vi "EOL station.vi"(0 "configuration file path":path caption="配置文件的路径", 1 "EOL station msic inf":T1) -> ()   [LabVIEW 2018]
uses:
  Ctl.xio/EOL station msic ctl.ctl
  SubVIS.xio/DataSocket/DataSocket_Tags.ctl
  Ctl.xio/part type.ctl
  SubVIS.xio/Creat Write List VI's/DefCtrl/Station.ctl
  <vilib>/Utility/file.llb/Read From Spreadsheet File (string).vi
  SubVIS.xio/DataSocket/Read PLC Vars/Read Bool Var.vi
  SubVIS.xio/DataSocket/Read PLC Vars/Read U32 Var.vi
  SubVIS.xio/DataSocket/Write PLC Vars/Write Bool Var in.vi
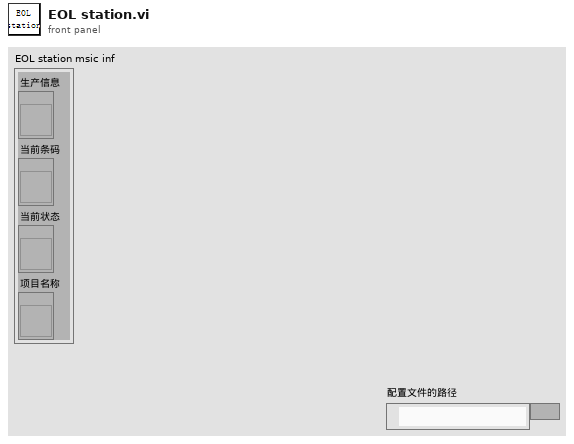
[diagram p1: front panel]
types:
  T1 = cluster{"生产信息":refnum<vi>, "当前条码":refnum<vi>, "当前状态":refnum<vi>, "项目名称":refnum<vi>}
  T2 = typedef "Station.ctl" = enum16{"粗切工位", "热处理工位", "精切工位", "PDF焊接工位", "打凹点预载力工位", "收卷工位", "EOL工位"}
  T3 = typedef "EOL station msic ctl.ctl" = cluster{"configuration file path":path, "DsOut":T4[], "Hopper car information":cluster{"Hopper car code":string, "Hopper car No":string, "plate No":string}, "pallet.produced number":i32, "SQL information":string, "Serial number":i32, "database path":path, "EOL station msic inf":cluster{"生产信息":refnum<vi>, "当前条码":refnum<vi>, "当前状态":refnum<vi>, "项目名称":refnum<vi>}, "part type":T5, "BarCode":string, "scanner resource name out":refnum<visa-resource-name>, "scanner coms":string, "Force value database":string[], "Force value buffer":dbl[], "SN":string, "print inf":string, "2Dcode inf":string, "Pass/Fail":bool}
  T4 = typedef "DataSocket_Tags.ctl" = cluster{"Ds ID":refnum<k13>, "Tag":string}
  T5 = typedef "part type.ctl" = cluster{"Part type":string, "Material code":string, "Part number":string, "Supplier code":string, "Line code":string, "Customer code":string, "Color code":string, "Upper limit":i32, "Temperature":string, "Tot time":string, "EOL stations":string}
  T6 = cluster{"Hopper car code":string, "Hopper car No":string, "plate No":string}
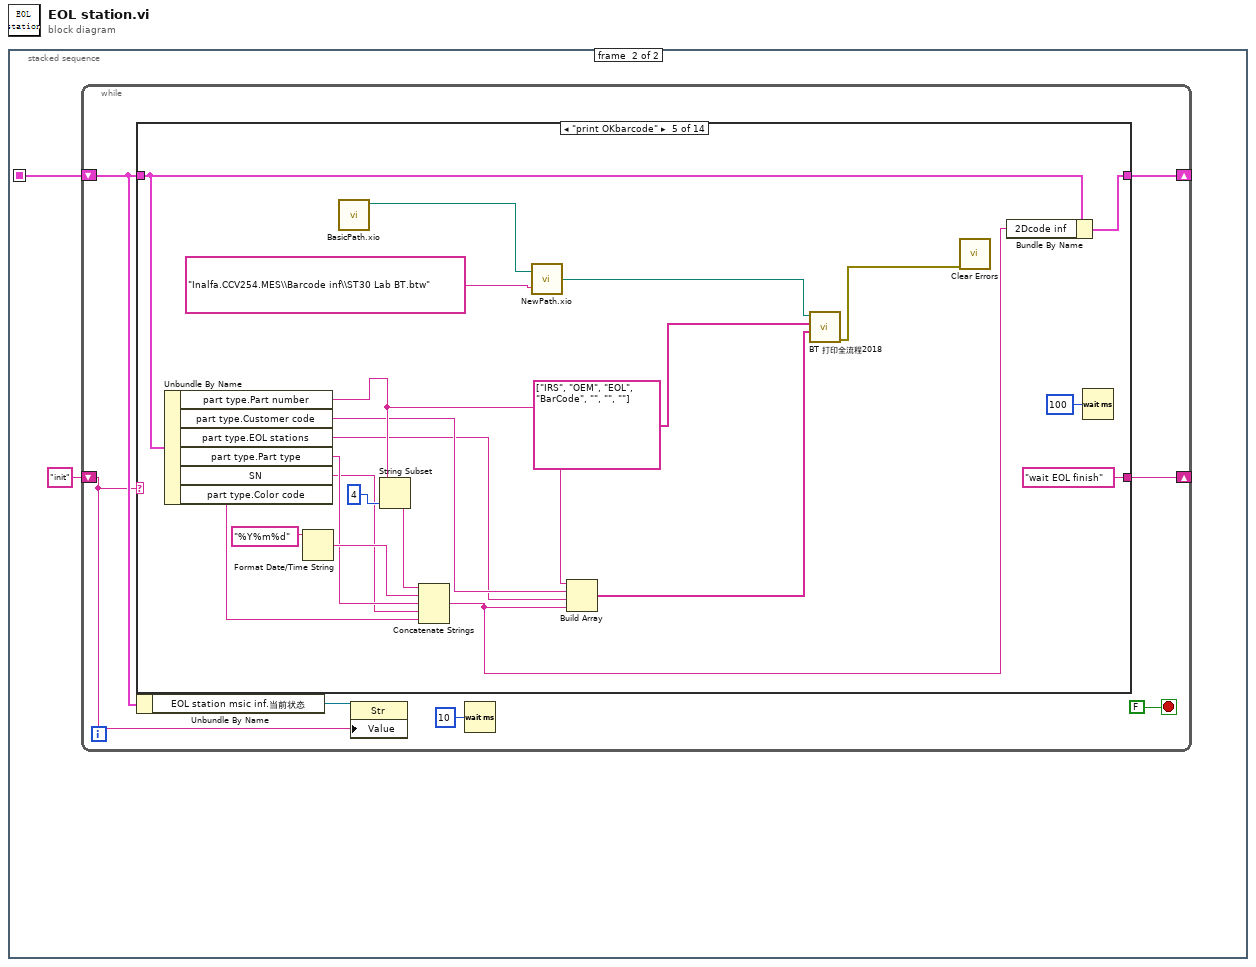
[diagram p0: block diagram]
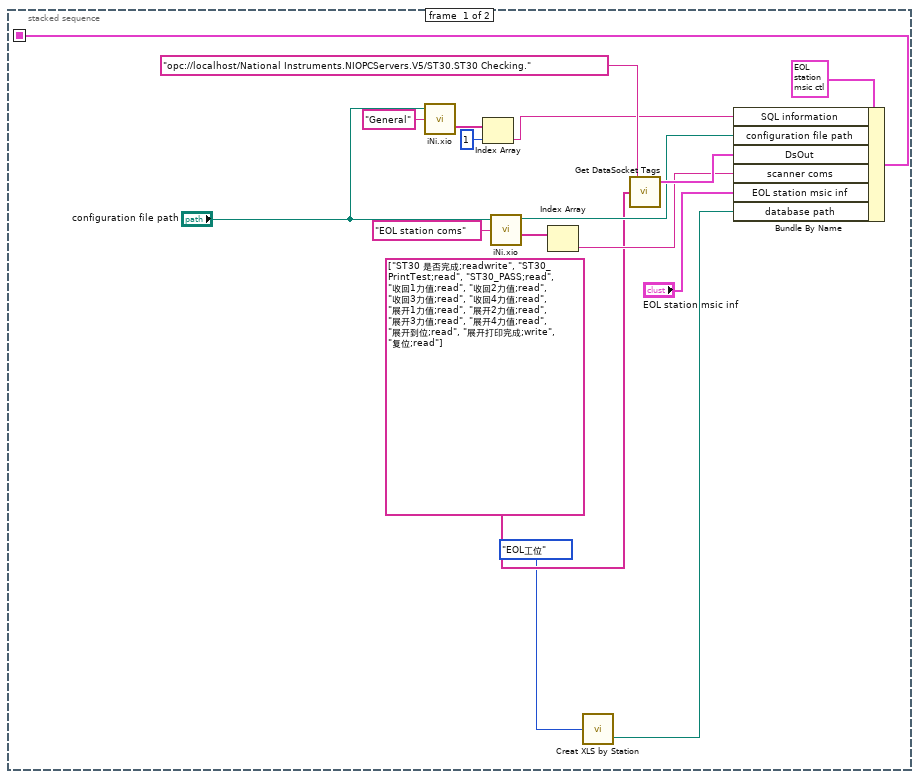
[diagram p2: hidden frame]
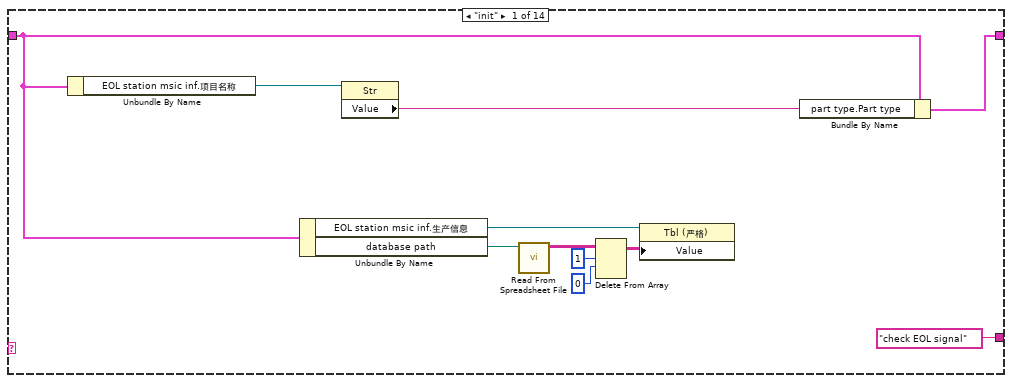
[diagram p3: hidden frame]
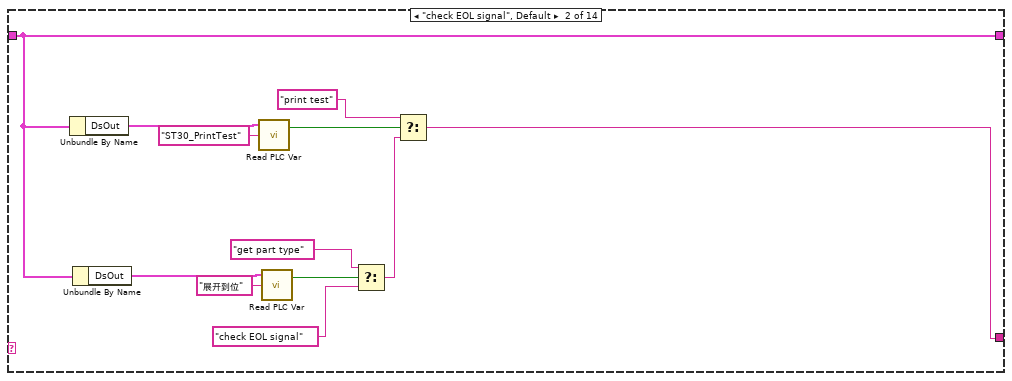
[diagram p4: hidden frame]
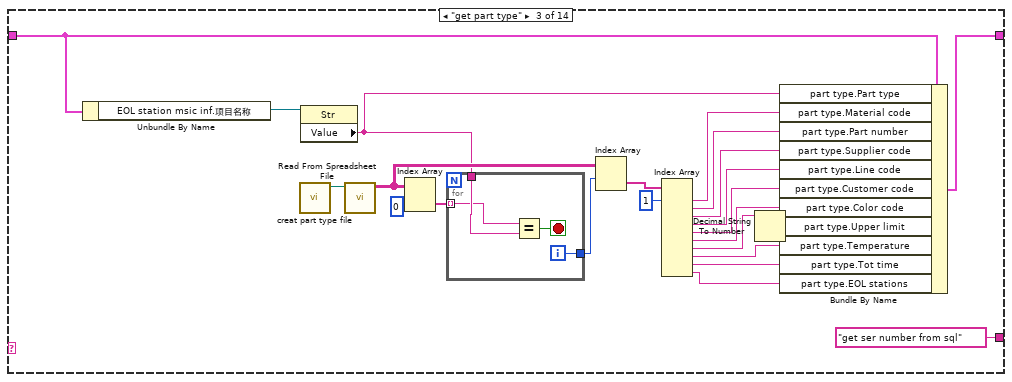
[diagram p5: hidden frame]
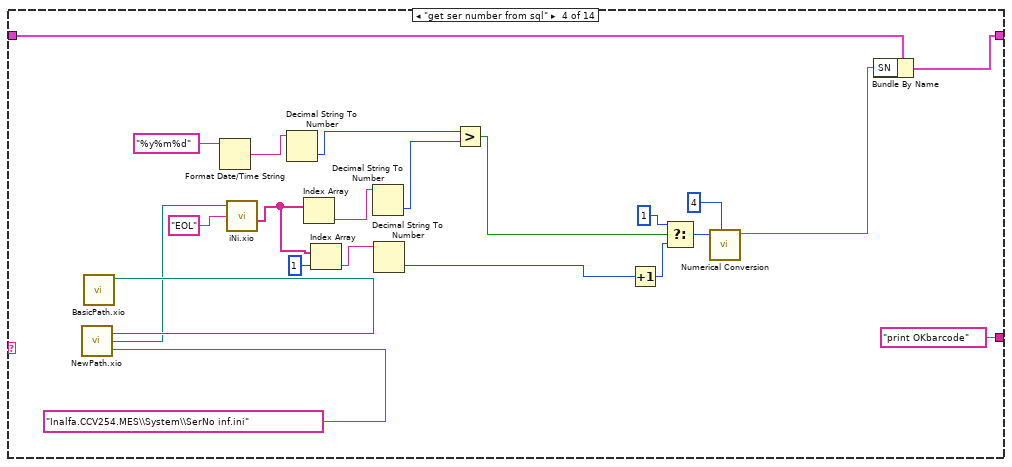
[diagram p6: hidden frame]
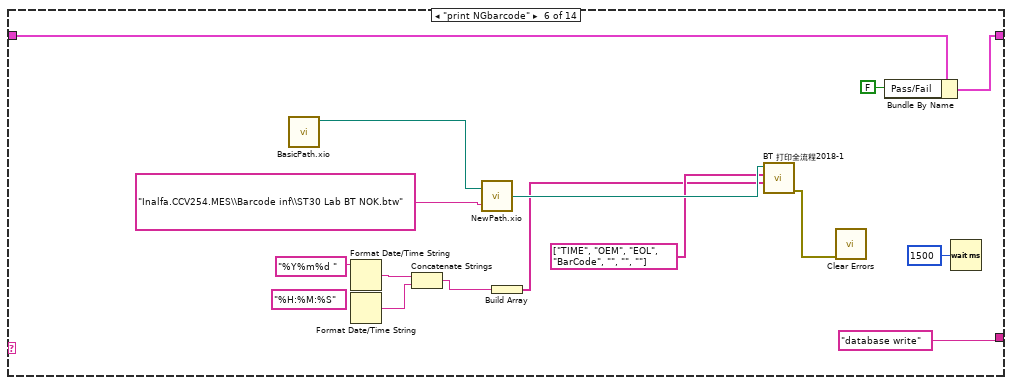
[diagram p7: hidden frame]
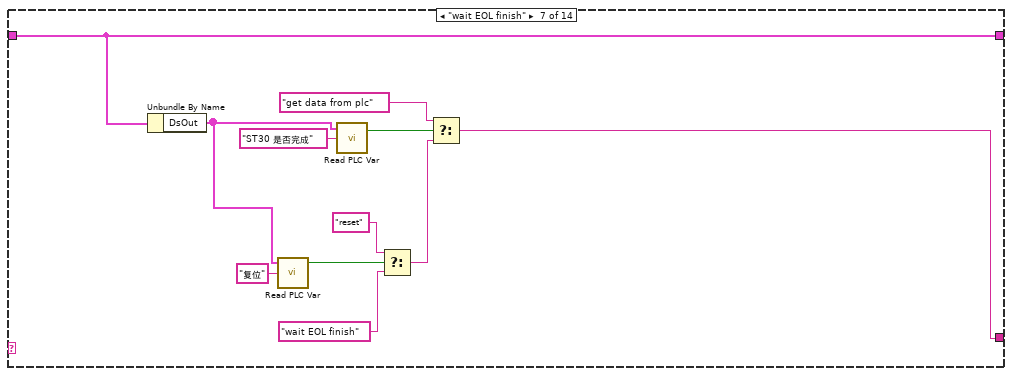
[diagram p8: hidden frame]
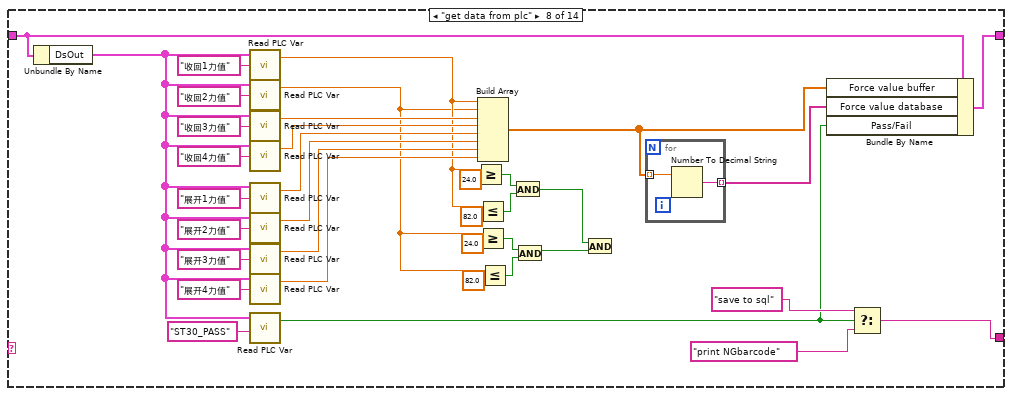
[diagram p9: hidden frame]
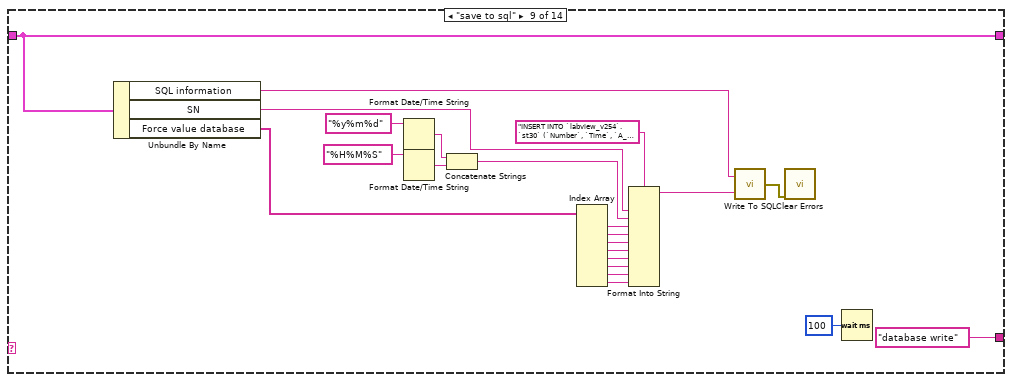
[diagram p10: hidden frame]
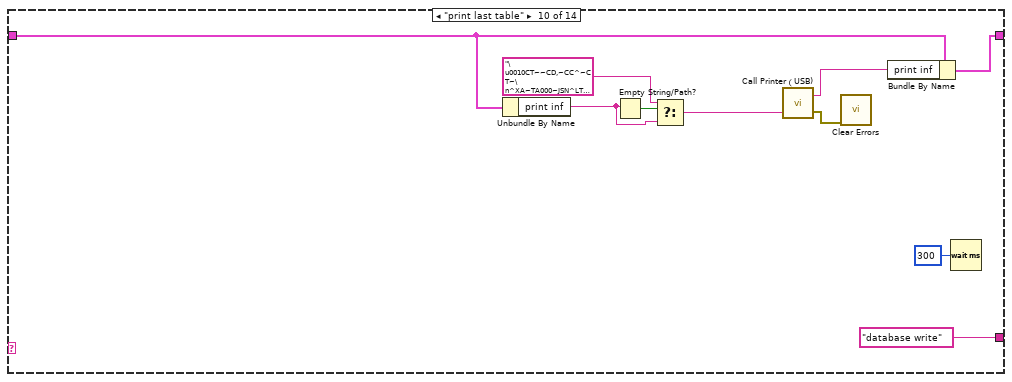
[diagram p11: hidden frame]
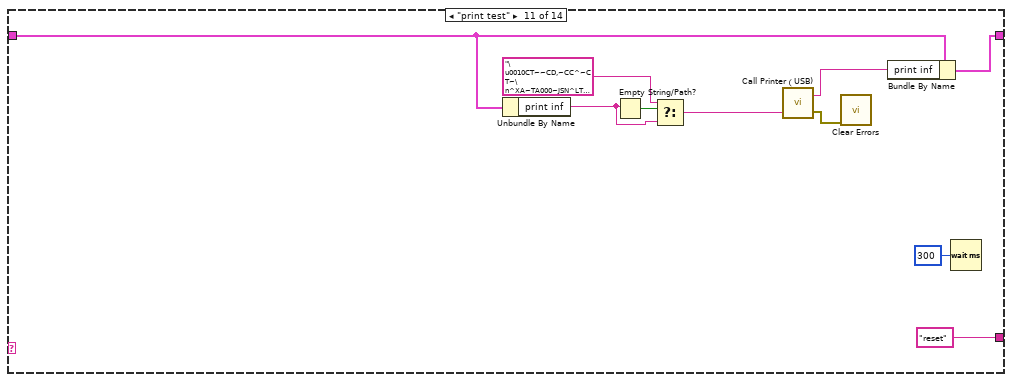
[diagram p12: hidden frame]
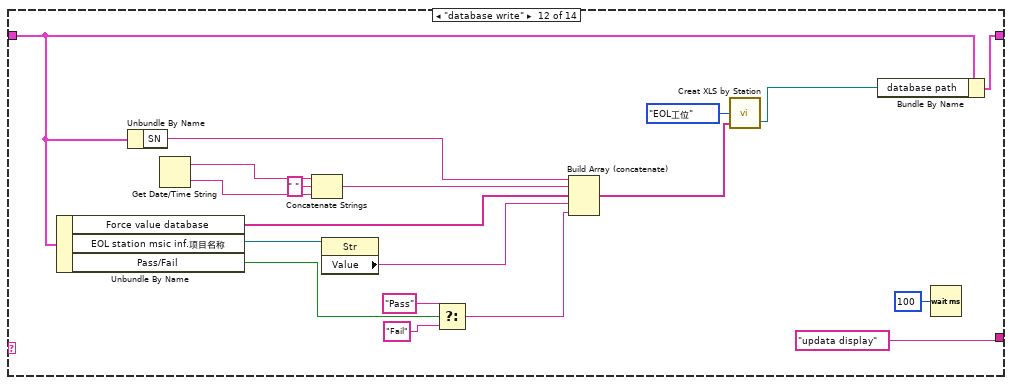
[diagram p13: hidden frame]
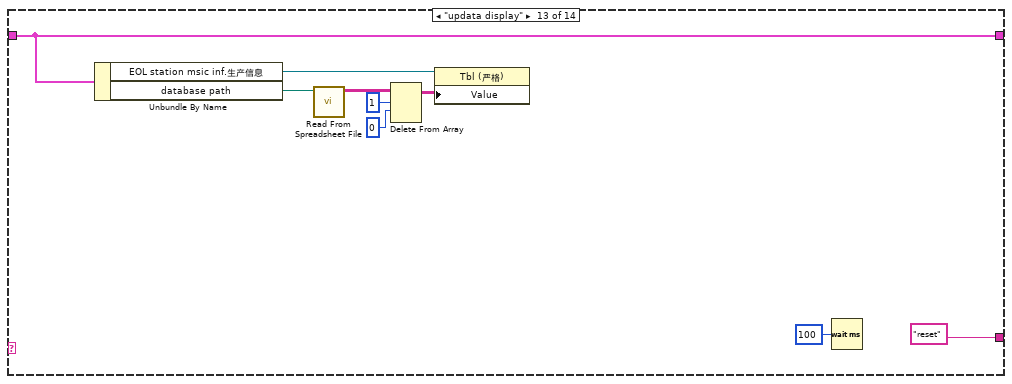
[diagram p14: hidden frame]
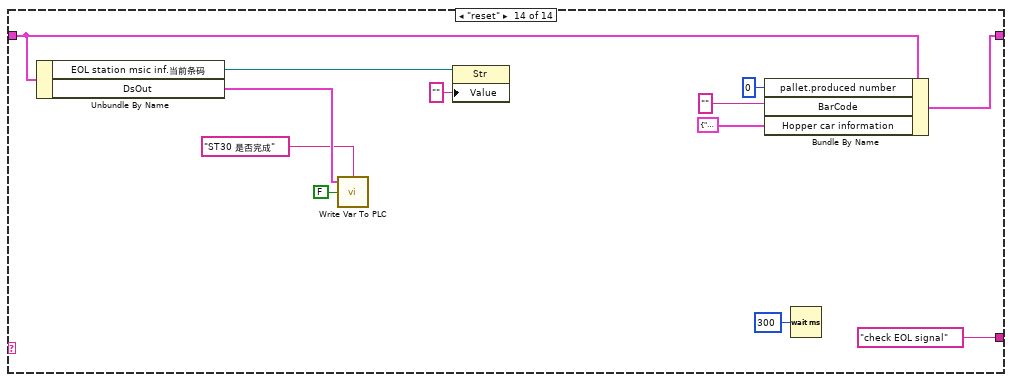
[diagram p15: hidden frame]
diagram:
  n1 = stacked-sequence {
    seq-local: [w10 _] -> [_ w18]
    frame #0 {
      n2 = call "iNi.xio.vi"("configuration file path"="configuration file path", "Sections"="General") -> ("Values"=w5:string[])  [unwired: 1 in, 4 out]
      n3 = Index Array(array=w5, index=1 ("索引")) -> (element=w3:string)
      n4 = call "iNi.xio.vi"("configuration file path"="configuration file path", "Sections"="EOL station coms") -> ("configuration file path"=w16:path, "Values"=w14:string[])  [unwired: 1 in, 3 out]
      n5 = Index Array(array=w14) -> (element=w13:string)  [unwired: 1 in]
      n6 = call "Creat XLS by Station.vi"("staiton"=Station."EOL工位") -> ("new file path (Not A Path if cancelled)"=w1:path)  [unwired: 5 in]
      n7 = call "Get DataSocket Tags.vi"("All Tags"=string[] ["ST30 是否完成;readwrite", "ST30_PrintTest;read", "ST30_PASS;read", "收回1力值;read", "收回2力值;read", "收回3力值;read", "收回4力值;read", "展开1力值;read", "展开2力值;read", "展开3力值;read", "展开4力值;read", "展开到位;read", "展开打印完成;write", "复位;read"], "URL"="opc://localhost/National Instruments.NIOPCServers.V5/ST30.ST30 Checking.") -> ("DsOut"=w17:T4[])  [unwired: 3 in]
      n8 = Bundle By Name(cluster=T3 {"configuration file path"=path "", "DsOut"=[], "Hopper car information"={"Hopper car code"="", "Hopper car No"="", "plate No"=""}, "pallet.produced number"=0, "SQL information"="", "Serial number"=0, "database path"=path "", "EOL station msic inf"={"生产信息"=refnum, "当前条码"=refnum, "当前状态"=refnum, "项目名称"=refnum}, "part type"={"Part type"="", "Material code"="", "Part number"="", "Supplier code"="", "Line code"="", "Customer code"="", "Color code"="", "Upper limit"=0, "Temperature"="", "Tot time"="", "EOL stations"=""}, "BarCode"="", "scanner resource name out"="", "scanner coms"="", "Force value database"=[], "Force value buffer"=[], "SN"="", "print inf"="", "2Dcode inf"="", "Pass/Fail"=FALSE} ("PDF Welding msic ctl"), "SQL information"=w3, "configuration file path"=w16, "DsOut"=w17, "scanner coms"=w13, "EOL station msic inf"="EOL station msic inf", "database path"=w1) -> (w10:T3)
    }
    frame #1 {
      n9 = while {
        shift-right: [w26] -> _
        shift-left: w18 -> [w21]
        shift-right: [w25] -> _
        shift-left: "init" ("event") -> [w20]
        stop <- FALSE stop-if-true
        n10 = case shown="\"print OKbarcode\"" w20 {
          tunnel: w21 -> [w27 w42 w71 w90 w113 w133 w142 w173 w186 w211 w221 w236 w251 w260]
          tunnel: [w37 w42 w50 w93 w116 w132 w142 w172 w186 w214 w224 w244 w251 w264] -> w26
          tunnel: ["check EOL signal" w38 "get ser number from sql" ("f") "print OKbarcode" ("f") "wait EOL finish" ("f") "database write" ("f") w141 w164 "database write" ("f") "database write" ("f") "reset" ("f") "updata display" ("f") "reset" ("f") "check EOL signal" ("f")] -> w25
          frame "init" {
            n11 = Unbundle By Name(w27) -> ("EOL station msic inf.项目名称"=w36:refnum<vi>)
            n12 = Unbundle By Name(w27) -> ("EOL station msic inf.生产信息"=w33:refnum<vi>, "database path"=w32:path)
            n13 = property class="Str"(reference=w36) -> ("Value"=w35:string)  [unwired: 1 in, 2 out]
            n14 = call-poly <vilib>:"Read From Spreadsheet File.vi"("file path (dialog if empty)"=w32) -> ("all rows"=w31:string[][])  [unwired: 6 in, 4 out]
            n15 = Delete From Array(array=w31, length=1 ("长度"), index (row)=0 ("索引 (行)")) -> (array with subset deleted=w28:string[][])  [unwired: 1 in, 1 out]
            n16 = property class="Tbl (严格)"(reference=w33, "Value"=w28) -> ()  [unwired: 1 in, 2 out]
            n17 = Bundle By Name(cluster=w27, "part type.Part type"=w35) -> (w37:T3)
          }
          frame "check EOL signal", Default {
            n18 = Unbundle By Name(w42) -> ("DsOut"=w43:T4[])
            n19 = Unbundle By Name(w42) -> ("DsOut"=w49:T4[])
            n20 = call-poly "Read PLC Var.vi"("Tag IN"="ST30_PrintTest", "Ds PLCTags IN"=w43) -> ("Bool Var out"=w41:bool)  [unwired: 1 in, 1 out]
            n21 = call-poly "Read PLC Var.vi"("Tag IN"="展开到位", "Ds PLCTags IN"=w49) -> ("Bool Var out"=w47:bool)  [unwired: 1 in, 1 out]
            n22 = Select(t="get part type" ("f"), s=w47, f="check EOL signal") -> (s? t:f=w40:string)
            n23 = Select(t="print test" ("f"), s=w41, f=w40) -> (s? t:f=w38:string)
          }
          frame "get part type" {
            n24 = Unbundle By Name(w71) -> ("EOL station msic inf.项目名称"=w72:refnum<vi>)
            n25 = call "creat part type file.vi"() -> ("new file path (Not A Path if cancelled)"=w65:path)  [unwired: 11 in]
            n26 = property class="Str"(reference=w72) -> ("Value"=w64:string)  [unwired: 1 in, 2 out]
            n27 = call-poly <vilib>:"Read From Spreadsheet File.vi"("file path (dialog if empty)"=w65) -> ("all rows"=w68:string[][])  [unwired: 6 in, 4 out]
            n28 = Index Array(array=w68, index (col)=0 ("禁用的索引 (列)")) -> (element=w69:string[])  [unwired: 1 in]
            n29 = for {
              tunnel: w69 -> [w73] mode=indexing
              tunnel: [w75] -> w67
              tunnel: w64 -> [w74]
              i -> [w75]
              stop <- w76 stop-if-true
              n30 = Equal?(x=w73, y=w74) -> (x = y?=w76:bool)
            }
            n31 = Index Array(array=w68, index (row)=w67) -> (element=w66:string[])  [unwired: 1 in]
            n32 = Index Array(array=w66, index #1=1 ("索引")) -> (element #1=w61:string, element #2=w60:string, element #3=w59:string, element #4=w58:string, element #5=w56:string, element #6=w57:string, element #7=w54:string, element #8=w53:string, element #9=w52:string, element #10=w51:string)  [unwired: 9 in]
            n33 = Decimal String To Number(string=w54) -> (number=w55:i32)  [unwired: 2 in, 1 out]
            n34 = Bundle By Name(cluster=w71, "part type.Part type"=w64, "part type.Material code"=w61, "part type.Part number"=w60, "part type.Supplier code"=w59, "part type.Line code"=w58, "part type.Customer code"=w56, "part type.Color code"=w57, "part type.Upper limit"=w55, "part type.Temperature"=w53, "part type.Tot time"=w52, "part type.EOL stations"=w51) -> (w50:T3)
          }
          frame "get ser number from sql" {
            n35 = call "BasicPath.xio.vi"() -> ("stripped path"=w88:path)  [unwired: 10 in, 1 out]
            n36 = call "NewPath.xio.vi"("Append path"="Inalfa.CCV254.MES\\System\\SerNo inf.ini", "Basic path"=w88) -> ("New path"=w85:path)
            n37 = Format Date/Time String(time format string (%c)="%y%m%d" ("时间格式字符串(%c)")) -> (date/time string=w82:string)  [unwired: 2 in]
            n38 = call "iNi.xio.vi"("configuration file path"=w85, "Sections"="EOL") -> ("Values"=w83:string[])  [unwired: 1 in, 4 out]
            n39 = Decimal String To Number(string=w82) -> (number=w81:i32)  [unwired: 2 in, 1 out]
            n40 = Index Array(array=w83) -> (element=w80:string)  [unwired: 1 in]
            n41 = Index Array(array=w83, index=1 ("索引")) -> (element=w77:string)
            n42 = Decimal String To Number(string=w80) -> (number=w79:i32)  [unwired: 2 in, 1 out]
            n43 = Decimal String To Number(string=w77) -> (number=w95:i32)  [unwired: 2 in, 1 out]
            n44 = Greater?(x=w81, y=w79) -> (0:w78:bool)
            n45 = Increment(x=w95) -> (x+1=w94:i32)
            n46 = Select(t=1, s=w78, f=w94) -> (s? t:f=w96:i32)
            n47 = call "Numerical Conversion.vi"("width"=4, "num"=w96) -> ("字符串"=w92:string)  [unwired: 9 in]
            n48 = Bundle By Name(cluster=w90, "SN"=w92) -> (w93:T3)
          }
          frame "print OKbarcode" {
            n49 = Unbundle By Name(w113) -> ("part type.Part number"=w107:string, "part type.Customer code"=w106:string, "part type.EOL stations"=w105:string, "part type.Part type"=w110:string, "SN"=w109:string, "part type.Color code"=w108:string)
            n50 = Format Date/Time String(time format string (%c)="%Y%m%d" ("时间格式字符串(%c)")) -> (date/time string=w117:string)  [unwired: 2 in]
            n51 = call "BasicPath.xio.vi"() -> ("stripped path"=w104:path)  [unwired: 10 in, 1 out]
            n52 = String Subset(string=w107, length (rest)=4 ("偏移量(0)")) -> (substring=w112:string)  [unwired: 1 in]
            n53 = Concatenate Strings(w112, w117, w110, w109, w108) -> (w115:string)
            n54 = call "NewPath.xio.vi"("Append path"="Inalfa.CCV254.MES\\Barcode inf\\ST30 Lab BT.btw", "Basic path"=w104) -> ("New path"=w103:path)
            n55 = Build Array(w107, w106, w105, w115) -> (w100:string[])
            n56 = call "BT 打印全流程2018.vi"("文件路径"=w103, "BT 具名数据源名称"=string[] ["IRS", "OEM", "EOL", "BarCode", "", "", ""], "输入内容"=w100) -> ("error out"=w99:errorcluster)  [unwired: 7 in]
            n57 = call <vilib>:"Clear Errors.vi"("error in (no error)"=w99) -> ()  [unwired: 5 in, 2 out]
            n58 = Bundle By Name(cluster=w113, "2Dcode inf"=w115) -> (w116:T3)
            n59 = Wait (ms)(milliseconds to wait=u32 100 ("等待时间（毫秒）")) -> ()  [unwired: 1 out]
          }
          frame "print NGbarcode" {
            (unwired) "%H:%M:%S" ("时间格式字符串(%c)")
            n60 = call "BasicPath.xio.vi"() -> ("stripped path"=w126:path)  [unwired: 10 in, 1 out]
            n61 = Format Date/Time String(time format string (%c)="%Y%m%d " ("时间格式字符串(%c)")) -> (date/time string=w131:string)  [unwired: 2 in]
            n62 = Format Date/Time String() -> (date/time string=w130:string)  [unwired: 3 in]
            n63 = Concatenate Strings(w131, w130) -> (w124:string)
            n64 = call "NewPath.xio.vi"("Append path"="Inalfa.CCV254.MES\\Barcode inf\\ST30 Lab BT NOK.btw", "Basic path"=w126) -> ("New path"=w123:path)
            n65 = Build Array(w124) -> (w121:string[])
            n66 = call "BT 打印全流程2018-1.vi"("文件路径"=w123, "BT 具名数据源名称"=string[] ["TIME", "OEM", "EOL", "BarCode", "", "", ""], "输入内容"=w121) -> ("error out"=w120:errorcluster)  [unwired: 7 in]
            n67 = call <vilib>:"Clear Errors.vi"("error in (no error)"=w120) -> ()  [unwired: 5 in, 2 out]
            n68 = Bundle By Name(cluster=w133, "Pass/Fail"=FALSE) -> (w132:T3)
            n69 = Wait (ms)(milliseconds to wait=u32 1500 ("等待时间（毫秒）")) -> ()  [unwired: 1 out]
          }
          frame "wait EOL finish" {
            n70 = Unbundle By Name(w142) -> ("DsOut"=w139:T4[])
            n71 = call-poly "Read PLC Var.vi"("Tag IN"="复位", "Ds PLCTags IN"=w139) -> ("Bool Var out"=w138:bool)  [unwired: 1 in, 1 out]
            n72 = call-poly "Read PLC Var.vi"("Tag IN"="ST30 是否完成", "Ds PLCTags IN"=w139) -> ("Bool Var out"=w144:bool)  [unwired: 1 in, 1 out]
            n73 = Select(t="reset" ("f"), s=w138, f="wait EOL finish") -> (s? t:f=w135:string)
            n74 = Select(t="get data from plc" ("f"), s=w144, f=w135) -> (s? t:f=w141:string)
          }
          frame "get data from plc" {
            n75 = Unbundle By Name(w173) -> ("DsOut"=w149:T4[])
            n76 = call-poly "Read PLC Var.vi"("Tag IN"="收回1力值", "Ds PLCTags IN"=w149) -> ("U32 Var out"=w160:dbl)  [unwired: 1 in, 1 out]
            n77 = call-poly "Read PLC Var.vi"("Tag IN"="收回2力值", "Ds PLCTags IN"=w149) -> ("U32 Var out"=w152:dbl)  [unwired: 1 in, 1 out]
            n78 = call-poly "Read PLC Var.vi"("Tag IN"="收回3力值", "Ds PLCTags IN"=w149) -> ("U32 Var out"=w171:dbl)  [unwired: 1 in, 1 out]
            n79 = call-poly "Read PLC Var.vi"("Tag IN"="收回4力值", "Ds PLCTags IN"=w149) -> ("U32 Var out"=w170:dbl)  [unwired: 1 in, 1 out]
            n80 = call-poly "Read PLC Var.vi"("Tag IN"="展开1力值", "Ds PLCTags IN"=w149) -> ("U32 Var out"=w166:dbl)  [unwired: 1 in, 1 out]
            n81 = call-poly "Read PLC Var.vi"("Tag IN"="展开2力值", "Ds PLCTags IN"=w149) -> ("U32 Var out"=w169:dbl)  [unwired: 1 in, 1 out]
            n82 = call-poly "Read PLC Var.vi"("Tag IN"="展开3力值", "Ds PLCTags IN"=w149) -> ("U32 Var out"=w168:dbl)  [unwired: 1 in, 1 out]
            n83 = call-poly "Read PLC Var.vi"("Tag IN"="展开4力值", "Ds PLCTags IN"=w149) -> ("U32 Var out"=w167:dbl)  [unwired: 1 in, 1 out]
            n84 = call-poly "Read PLC Var.vi"("Tag IN"="ST30_PASS", "Ds PLCTags IN"=w149) -> ("Bool Var out"=w146:bool)  [unwired: 1 in, 1 out]
            n85 = Greater Or Equal?(x=w160, y=24.0) -> (x >= y?=w157:bool)
            n86 = Build Array(w160, w152, w171, w170, w166, w169, w168, w167) -> (w163:dbl[])
            n87 = Less Or Equal?(x=w160, y=82.0) -> (x <= y?=w158:bool)
            n88 = Greater Or Equal?(x=w152, y=24.0) -> (x >= y?=w156:bool)
            n89 = Less Or Equal?(x=w152, y=82.0) -> (x <= y?=w155:bool)
            n90 = And(x=w157, y=w158) -> (x .and. y?=w150:bool)
            n91 = And(x=w156, y=w155) -> (x .and. y?=w151:bool)
            n92 = And(x=w150, y=w151) -> ()  [unwired: 1 out]
            n93 = for {
              tunnel: w163 -> [w183] mode=indexing
              tunnel: [w182] -> w162 mode=indexing
              n94 = Number To Decimal String(number=w183) -> (decimal integer string=w182:string)  [unwired: 1 in]
            }
            n95 = Bundle By Name(cluster=w173, "Force value buffer"=w163, "Force value database"=w162, "Pass/Fail"=w146) -> (w172:T3)
            n96 = Select(t="save to sql" ("f"), s=w146, f="print NGbarcode") -> (s? t:f=w164:string)
          }
          frame "save to sql" {
            n97 = Unbundle By Name(w186) -> ("SQL information"=w188:string, "SN"=w200:string, "Force value database"=w199:string[])
            n98 = Format Date/Time String(time format string (%c)="%y%m%d" ("时间格式字符串(%c)")) -> (date/time string=w203:string)  [unwired: 2 in]
            n99 = Format Date/Time String(time format string (%c)="%H%M%S" ("时间格式字符串(%c)")) -> (date/time string=w204:string)  [unwired: 2 in]
            n100 = Concatenate Strings(w203, w204) -> (w201:string)
            n101 = Index Array(array=w199) -> (element #1=w198:string, element #2=w197:string, element #3=w196:string, element #4=w195:string, element #5=w194:string, element #6=w193:string, element #7=w192:string, element #8=w191:string)  [unwired: 8 in]
            n102 = Format Into String(format string="INSERT INTO `labview_v254`.`st30` (`Number`, `Time`, `A_Data1`, `A_Data2`, `A_Data3`, `A_Data4`, `B_Data1`, `B_Data2`, `B_Data3`, `B_Data4`) VALUES ('%s', '%s', '%s', '%s', '%s', '%s', '%s', '%s', '%s', '%s');" ("初始字符串"), w200, w201, w198, w197, w196, w195, w194, w193, w192, w191) -> (resulting string=w189:string)  [unwired: 2 in, 1 out]
            n103 = call "Write To SQL.vi"("SQL query"=w189, "connection information"=w188) -> ("error out"=w187:errorcluster)
            n104 = call <vilib>:"Clear Errors.vi"("error in (no error)"=w187) -> ()  [unwired: 5 in, 2 out]
            n105 = Wait (ms)(milliseconds to wait=u32 100 ("等待时间（毫秒）")) -> ()  [unwired: 1 out]
          }
          frame "print last table" {
            n106 = Unbundle By Name(w211) -> ("print inf"=w208:string)
            n107 = Empty String/Path?(string/path=w208) -> (empty?=w210:bool)
            n108 = Select(t="\u0010CT~~CD,~CC^~CT~\n^XA~TA000~JSN^LT0^MNW^MTT^PON^PMN^LH0,0^JMA^PR5,5~SD15^JUS^LRN^CI0^XZ\n~DG000.GRF,00768,024,\n,::I07,I0780I0J8H0LA80H0E0I0380E,I0380I0IFE007FJF8001E0I0181C,02ABAA800EAAE002H2E228003F0I038380I0F0,07FIFC00C0060I01C0J0H3J0101FF80070,H0K8H0E00E0I01C0J0FBC0H0383AF800F0,H0701C0H0C0060I01C0J0E1C0017D7870H070,H0781E0H0E00E0I0380I03E0F003FHF870H0F0,H0301C0H0C0060I0780I0380780031DC70H070,H03C380H0IFE0I0F9C0H0F803E0078CEE0H0F0,J030P01FDE001E0H0FC07C07C0H070,0FJFE0N03B8F007BFHF3C0FE0380H0E0,07FIFE0N071870071J1H07F07E0H070,0E0K0HFEFFE00FB83C020L0HFBEFE00E0,070K0HFC7FE01C1C1E0M01F9F01E0060,0E0K0E0EE0E038380F003BHB803B9E00E0060,060K0C0C60607018070075H5C01907FF8,0E0K0E0EE0E0E0380200E001C03B838B8,0E0K0C0C6060H01C0I07001C01187018,0E0K0E0EE0E0H0380I0E001C00383038,1C0K0C0C6060H0180I07001C001070180070,1E0K0HFEFFE0H0380I0FAABC0038783800F0,1C0K0HFC7FE0H01C0I07FHFC00187D7800F0,380K0E0EE060H0380I0E003C00383AB8,30L040440J0180I07001C00107018,X080I0A0H0800282828,,::^XA\n^MMT\n^PW719\n^LL0096\n^LS0\n^FT166,88^A0N,20,21^FH\\^FDZX^FS\n^FT416,64^XG000.GRF,1,1^FS\n^FT78,88^A0N,20,21^FH\\^FDSerial nr:^FS\n^FT142,44^A0N,28,28^FH\\^FDNok^FS\n^PQ1,0,1,Y^XZ\n^XA^ID000.GRF^FS^XZ", s=w210, f=w208) -> (s? t:f=w207:string)
            n109 = call "Call Printer（USB).vi"("写入缓冲区"=w207) -> ("error out"=w213:errorcluster, "Last P"=w215:string)  [unwired: 1 in]
            n110 = call <vilib>:"Clear Errors.vi"("error in (no error)"=w213) -> ()  [unwired: 5 in, 2 out]
            n111 = Bundle By Name(cluster=w211, "print inf"=w215) -> (w214:T3)
            n112 = Wait (ms)(milliseconds to wait=u32 300 ("等待时间（毫秒）")) -> ()  [unwired: 1 out]
          }
          frame "print test" {
            n113 = Unbundle By Name(w221) -> ("print inf"=w218:string)
            n114 = Empty String/Path?(string/path=w218) -> (empty?=w220:bool)
            n115 = Select(t="\u0010CT~~CD,~CC^~CT~\n^XA~TA000~JSN^LT0^MNW^MTT^PON^PMN^LH0,0^JMA^PR5,5~SD15^JUS^LRN^CI0^XZ\n~DG000.GRF,00768,024,\n,::I07,I0780I0J8H0LA80H0E0I0380E,I0380I0IFE007FJF8001E0I0181C,02ABAA800EAAE002H2E228003F0I038380I0F0,07FIFC00C0060I01C0J0H3J0101FF80070,H0K8H0E00E0I01C0J0FBC0H0383AF800F0,H0701C0H0C0060I01C0J0E1C0017D7870H070,H0781E0H0E00E0I0380I03E0F003FHF870H0F0,H0301C0H0C0060I0780I0380780031DC70H070,H03C380H0IFE0I0F9C0H0F803E0078CEE0H0F0,J030P01FDE001E0H0FC07C07C0H070,0FJFE0N03B8F007BFHF3C0FE0380H0E0,07FIFE0N071870071J1H07F07E0H070,0E0K0HFEFFE00FB83C020L0HFBEFE00E0,070K0HFC7FE01C1C1E0M01F9F01E0060,0E0K0E0EE0E038380F003BHB803B9E00E0060,060K0C0C60607018070075H5C01907FF8,0E0K0E0EE0E0E0380200E001C03B838B8,0E0K0C0C6060H01C0I07001C01187018,0E0K0E0EE0E0H0380I0E001C00383038,1C0K0C0C6060H0180I07001C001070180070,1E0K0HFEFFE0H0380I0FAABC0038783800F0,1C0K0HFC7FE0H01C0I07FHFC00187D7800F0,380K0E0EE060H0380I0E003C00383AB8,30L040440J0180I07001C00107018,X080I0A0H0800282828,,::^XA\n^MMT\n^PW719\n^LL0096\n^LS0\n^FT166,88^A0N,20,21^FH\\^FDZX^FS\n^FT416,64^XG000.GRF,1,1^FS\n^FT78,88^A0N,20,21^FH\\^FDSerial nr:^FS\n^FT142,44^A0N,28,28^FH\\^FDNok^FS\n^PQ1,0,1,Y^XZ\n^XA^ID000.GRF^FS^XZ", s=w220, f=w218) -> (s? t:f=w217:string)
            n116 = call "Call Printer（USB).vi"("写入缓冲区"=w217) -> ("error out"=w223:errorcluster, "Last P"=w225:string)  [unwired: 1 in]
            n117 = call <vilib>:"Clear Errors.vi"("error in (no error)"=w223) -> ()  [unwired: 5 in, 2 out]
            n118 = Bundle By Name(cluster=w221, "print inf"=w225) -> (w224:T3)
            n119 = Wait (ms)(milliseconds to wait=u32 300 ("等待时间（毫秒）")) -> ()  [unwired: 1 out]
          }
          frame "database write" {
            n120 = Unbundle By Name(w236) -> ("Force value database"=w237:string[], "EOL station msic inf.项目名称"=w235:refnum<vi>, "Pass/Fail"=w232:bool)
            n121 = Unbundle By Name(w236) -> ("SN"=w243:string)
            n122 = Get Date/Time String() -> (date string=w240:string, time string=w239:string)  [unwired: 3 in]
            n123 = Concatenate Strings(w240, " " ("字符串"), w239) -> (w242:string)
            n124 = property class="Str"(reference=w235) -> ("Value"=w234:string)  [unwired: 1 in, 2 out]
            n125 = Select(t="Pass", s=w232, f="Fail") -> (s? t:f=w229:string)
            n126 = Build Array (concatenate)(w243, w242, w237, w234, w229) -> (w227:string[])
            n127 = call "Creat XLS by Station.vi"("staiton"=Station."EOL工位", "data in"=w227) -> ("new file path (Not A Path if cancelled)"=w226:path)  [unwired: 4 in]
            n128 = Bundle By Name(cluster=w236, "database path"=w226) -> (w244:T3)
            n129 = Wait (ms)(milliseconds to wait=u32 100 ("等待时间（毫秒）")) -> ()  [unwired: 1 out]
          }
          frame "updata display" {
            n130 = Unbundle By Name(w251) -> ("EOL station msic inf.生产信息"=w253:refnum<vi>, "database path"=w252:path)
            n131 = call-poly <vilib>:"Read From Spreadsheet File.vi"("file path (dialog if empty)"=w252) -> ("all rows"=w250:string[][])  [unwired: 6 in, 4 out]
            n132 = Delete From Array(array=w250, length=1 ("长度"), index (row)=0 ("索引 (行)")) -> (array with subset deleted=w247:string[][])  [unwired: 1 in, 1 out]
            n133 = property class="Tbl (严格)"(reference=w253, "Value"=w247) -> ()  [unwired: 1 in, 2 out]
            n134 = Wait (ms)(milliseconds to wait=u32 100 ("等待时间（毫秒）")) -> ()  [unwired: 1 out]
          }
          frame "reset" {
            n135 = Unbundle By Name(w260) -> ("EOL station msic inf.当前条码"=w259:refnum<vi>, "DsOut"=w256:T4[])
            n136 = call-poly "Write Var To PLC.vi"("Tag IN"="ST30 是否完成", "Bool Var in"=FALSE, "Ds PLCTags IN"=w256) -> ()  [unwired: 1 in, 2 out]
            n137 = property class="Str"(reference=w259, "Value"="" ("值")) -> ()  [unwired: 1 in, 2 out]
            n138 = Bundle By Name(cluster=w260, "pallet.produced number"=0, "BarCode"="", "Hopper car information"=T6 {"Hopper car code"="", "Hopper car No"="", "plate No"=""}) -> (w264:T3)
            n139 = Wait (ms)(milliseconds to wait=u32 300 ("等待时间（毫秒）")) -> ()  [unwired: 1 out]
          }
        }
        n140 = Unbundle By Name(w21) -> ("EOL station msic inf.当前状态"=w22:refnum<vi>)
        n141 = property class="Str"(reference=w22, "Value"=w20) -> ()  [unwired: 1 in, 2 out]
        n142 = Wait (ms)(milliseconds to wait=u32 10 ("等待时间（毫秒）")) -> ()  [unwired: 1 out]
      }
    }
  }
